vi "Configure CW Generation.vi"(0 "session in":T1[](array[typedef]) {"rx baseband session"."3630 session"."Address Space" items=["VXI/VME A16"=1, "VXI/VME A24"=2, "VXI/VME A32"=3, "VXI/VME A64"=4, "PXI Memory Allocations"=9, "PXI Configuration"=10, "PXI BAR0"=11, "PXI BAR1"=12, "PXI BAR2"=13, "PXI BAR3"=14, "PXI BAR4"=15, "PXI BAR5"=16]; "tx baseband session"."3610 session"."Address Space" items=["VXI/VME A16"=1, "VXI/VME A24"=2, "VXI/VME A32"=3, "VXI/VME A64"=4, "PXI Memory Allocations"=9, "PXI Configuration"=10, "PXI BAR0"=11, "PXI BAR1"=12, "PXI BAR2"=13, "PXI BAR3"=14, "PXI BAR4"=15, "PXI BAR5"=16]}, 5 "tone 1":cluster{"frequency (Hz)":dbl, "gain (dBFS)":dbl}={"frequency (Hz)"=0.0, "gain (dBFS)"=-inf} {"gain (dBFS)" format="%#_13g"; "frequency (Hz)" format="%#_13p"}, 7 "tone 2":cluster{"frequency (Hz)":dbl, "gain (dBFS)":dbl}={"frequency (Hz)"=0.0, "gain (dBFS)"=-inf} {"gain (dBFS)" format="%#_13g"; "frequency (Hz)" format="%#_13p"}, 9 "sample rate":dbl=3072000000.0 format="%#_13p", 11 "error in":errorcluster) -> (4 "session out":T1[](array[typedef]) {"rx baseband session"."3630 session"."Address Space" items=["VXI/VME A16"=1, "VXI/VME A24"=2, "VXI/VME A32"=3, "VXI/VME A64"=4, "PXI Memory Allocations"=9, "PXI Configuration"=10, "PXI BAR0"=11, "PXI BAR1"=12, "PXI BAR2"=13, "PXI BAR3"=14, "PXI BAR4"=15, "PXI BAR5"=16]; "tx baseband session"."3610 session"."Address Space" items=["VXI/VME A16"=1, "VXI/VME A24"=2, "VXI/VME A32"=3, "VXI/VME A64"=4, "PXI Memory Allocations"=9, "PXI Configuration"=10, "PXI BAR0"=11, "PXI BAR1"=12, "PXI BAR2"=13, "PXI BAR3"=14, "PXI BAR4"=15, "PXI BAR5"=16]}, 15 "error out":errorcluster)   [LabVIEW 2019]
uses:
  TypeDefs/Session.ctl
  <instrlib>/niMmWave/ni3620/Config/v1/Host/Public/High-Level/niMmWave Session.ctl
  <instrlib>/_niInstr/Register Bus/v0/Host/Public/Register Bus Session.ctl
  <instrlib>/_niInstr/Register Bus/v0/Host/Private/Session Data.ctl
  <instrlib>/niMmWave/ni3620/Config/v1/Host/Public/Typedefs/Board Information.ctl
  <instrlib>/niMmWave/ni3620/Config/v1/Host/Public/Typedefs/Hardware Revision.ctl
  <instrlib>/niMmWave/ni3620/Config/v1/Host/Public/Typedefs/Gain Mapping.ctl
  <instrlib>/niMmWave/ni3620/Config/v1/Host/Public/Typedefs/Correction Data.ctl
  <instrlib>/niMmWave/ni3620/Config/v1/Host/Public/Typedefs/Opera Characterization.ctl
  <instrlib>/niMmWave/ni3620/Config/v1/Host/Public/Corrections/Typedefs/Opera Characterization Main Header.ctl
  <instrlib>/niMmWave/ni3620/Config/v1/Host/Public/Corrections/Typedefs/Opera IF Board Information.ctl
  <instrlib>/niMmWave/ni3620/Config/v1/Host/Public/Corrections/Typedefs/Opera Characterization Instance Header.ctl
  <instrlib>/niMmWave/ni3620/Config/v1/Host/Public/Corrections/Typedefs/Opera Characterization Device Data Header.ctl
  <instrlib>/niMmWave/ni3620/Config/v1/Host/Public/Corrections/Typedefs/Opera LO Characterization Data Header.ctl
  <instrlib>/niMmWave/ni3620/Config/v1/Host/Public/Corrections/Typedefs/Opera IF Board Characterization Data Header.ctl
  <instrlib>/niMmWave/ni3620/Config/v1/Host/Public/Corrections/Typedefs/Opera Characterization Device Data.ctl
  <instrlib>/niMmWave/ni3620/Config/v1/Host/Public/Corrections/Typedefs/Opera LO2 Board Characterization Data.ctl
  <instrlib>/niMmWave/ni3620/Config/v1/Host/Public/Corrections/Typedefs/Opera LO Characterization Data.ctl
  <instrlib>/niMmWave/ni3620/Config/v1/Host/Public/Corrections/Typedefs/Opera IF Board Characterization Data.ctl
  <instrlib>/niMmWave/ni3620/Config/v1/Host/Public/Corrections/Typedefs/Opera IQ Impairment Data.ctl
  <instrlib>/niMmWave/ni3620/Config/v1/Host/Public/Typedefs/mmWave Adapter Session Data.ctl
  <instrlib>/niMmWave/ni3620/Config/v1/Host/Public/Typedefs/mmWave Adapter Data.ctl
  <instrlib>/niMmWave/ni3620/Config/v1/Host/Public/Typedefs/mmWave Adapter 2.ctl
  <instrlib>/niMmWave/ni3620/Config/v1/Shared/Typedefs/Subsystem ID.ctl
  <instrlib>/niMmWave/ni3620/Config/v1/Host/Public/Typedefs/mmWave Adapter Channel Information.ctl
  <instrlib>/niMmWave/ni3620/Config/v1/Host/Public/Typedefs/Temperature Coefficients.ctl
  <instrlib>/niMmWave/ni3620/Config/v1/Host/Public/Typedefs/mmWave Characterization.ctl
  <instrlib>/niMmWave/ni3620/Config/v1/Host/Public/Corrections/Typedefs/mmWave Characterization Main Header.ctl
  <instrlib>/niMmWave/ni3620/Config/v1/Host/Public/Corrections/Typedefs/mmWave Characterization Instance Header.ctl
  <instrlib>/niMmWave/ni3620/Config/v1/Host/Public/Typedefs/Session Cache.ctl
  <instrlib>/niMmWave/ni3620/Config/v1/Host/Public/Typedefs/LO2 settings cache.ctl
  <instrlib>/niMmWave/ni3620/Config/v1/Host/Public/Typedefs/LO2 source.ctl
  <instrlib>/niMmWave/ni3620/Config/v1/Host/Public/Typedefs/Desired and Coerced.ctl
  <instrlib>/niMmWave/ni3620/Config/v1/Host/Public/Typedefs/Export cache.ctl
  <instrlib>/niMmWave/ni3620/Config/v1/Host/Public/Typedefs/Path cache.ctl
  <instrlib>/niMmWave/ni3620/Config/v1/Host/Public/Typedefs/Daughterboard Type.ctl
  <instrlib>/niMmWave/ni3620/Config/v1/Host/Public/Typedefs/LO1 settings cache.ctl
  <instrlib>/niMmWave/ni3620/Config/v1/Host/Public/Typedefs/LO1 Source.ctl
  <instrlib>/niMmWave/ni3620/Config/v1/Host/Public/Typedefs/mmWave export cache.ctl
  <instrlib>/niMmWave/ni3620/Config/v1/Host/Private/Board/LO2/LO2 Board Configuration Cache.ctl
  <instrlib>/niMmWave/ni3620/Config/v1/Host/Public/Typedefs/reference clock routing settings.ctl
  <instrlib>/niMmWave/ni3620/Config/v1/Host/Public/Typedefs/LO2 routing settings.ctl
  <instrlib>/niMmWave/ni3620/Config/v1/Host/Private/Board/LO1/LO1 Board Configuration Cache.ctl
  <instrlib>/niMmWave/ni3620/Config/v1/Host/Public/Typedefs/LO1 source settings.ctl
  <instrlib>/niMmWave/ni3620/Config/v1/Host/Public/Typedefs/LO1 export settings.ctl
  <instrlib>/niMmWave/ni3620/Config/v1/Host/Public/Typedefs/LO1 mmWave settings.ctl
  TypeDefs/Tx Baseband Session.ctl
  <instrlib>/niMmWave/ni3610 and ni3630/controls/public/Main Settings.ctl
  <vilib>/Instr/_visa.llb/VISA Register Access Address Space.ctl
  <instrlib>/niMmWave/ni3610 and ni3630/controls/public/Register Adresses.ctl
  <instrlib>/niMmWave/ni3610 and ni3630/controls/public/Base Card Type.ctl
  <instrlib>/niMmWave/ni3610 and ni3630/controls/private/IQ Card Revision.ctl
  <instrlib>/niMmWave/ni3610 and ni3630/controls/public/Board Capability.ctl
  TypeDefs/Blank FPGA Reference.ctl
  TypeDefs/Rx Baseband Session.ctl
  TypeDefs/Hardware Configuration.ctl
  TypeDefs/Direction.ctl
  TypeDefs/Gain Ranging.ctl
  TypeDefs/PXI Trigger Bus Info.ctl
  TypeDefs/TX FPGA Reference.ctl
  <vilib>/Utility/error.llb/Error Cluster From Error Code.vi
  <vilib>/rvi/errors/niLvFpgaAdjustHostInterfaceError.vi
  <vilib>/rvi/interface/nirviReadWriteControl/nirviReadWriteControl.xnode
  mmWave HW Control/mmWave HW Control.lvlib
  NiFpgaLv.dll
  <vilib>/rvi/interface/Simulation/niFpgaSimulationCallBeginRW.vi
  <instrlib>/niMmWave/ni3620/Config/v1/Host/niMmWave Config v1 Host.lvlib
  <instrlib>/niMmWave/ni3620/Config/v1/Shared/niMmWave Config v1 Shared.lvlib
  <instrlib>/_niInstr/Register Bus/v0/Host/niInstr Register Bus v0 Host.lvlib
  <instrlib>/niMmWave/ni3610 and ni3630/ni3610_and_ni3630_Driver_Lib.lvlib
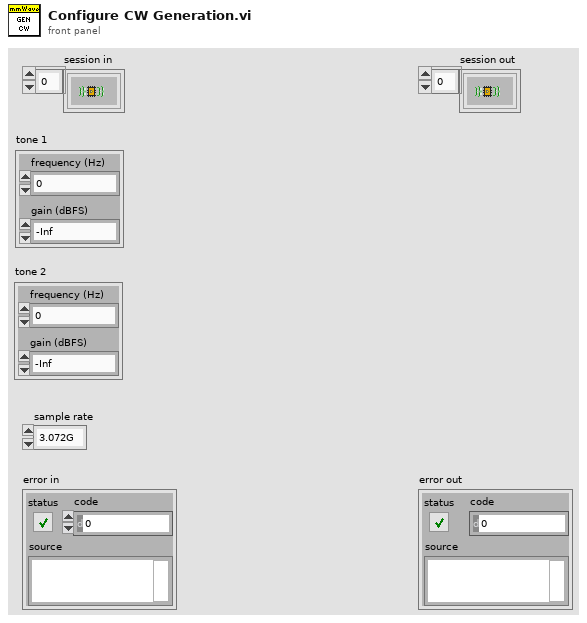
[diagram p1: front panel]
types:
  T1 = typedef "Session.ctl" = cluster{"3620 session":refnum<queue>, "tx baseband session":T2, "rx baseband session":T10, "tx gain (dB)":dbl, "rx gain (dB)":dbl, "hardware configuration":T11, "gain ranging":T13[], "pxi trigger bus information":T14}
  T2 = typedef "Tx Baseband Session.ctl" = cluster{"3610 session":T3, "7902 reference":T9}
  T3 = typedef "ni3610_and_ni3630_Driver_Lib.lvlib/Main Settings.ctl" = cluster{"VISA resource name":refnum<visa-resource-name>, "Address Space":T4, "window_offset":u32, "register_addresses":T5, "required_MM_fpga_version":cluster{"signature":u32, "hardware":u32, "current revision":u32, "oldest revision":u32}, "CPLD Oldest Compat Version ":cluster{"hardware":u32, "CPLD firmware":u32}, "MM_FPGA_image_location":string, "is_init":bool, "card_type":T6, "DacLmkConfigFileName":string, "AdcLmkConfigFileName":string, "AdcConfigFileName":string, "DacConfigFileName_RevA":string, "DacConfigFileName_RevB":string, "Mulde hardware revision":u8, "bypass DAC PLL\n":bool, "IQ Card Revision":T7, "board capability":T8}
  T4 = typedef "VISA Register Access Address Space.ctl" = u16
  T5 = typedef "ni3610_and_ni3630_Driver_Lib.lvlib/Register Adresses.ctl" = cluster{"MM based Registers":cluster{"Revision":u32, "OldestCompatRev":u32, "signature":u32, "scratch":u32, "LedControl":u32, "BoardHwRev":u32, "BoardControl":u32, "ThermalStatus":u32, "BasebandStatus":u32, "BasebandControl":u32, "BasebandAuxSetup":u32, "BasebandAuxStatus":u32, "LmkSyncOutSetup":u32, " AdcSyncOutSetup":u32, " InjSyncOutSetup":u32, " PxiTrig0OutSetup":u32, " PxiTrig1OutSetup":u32, " PxiTrig2OutSetup":u32, " PxiTrig3OutSetup":u32, " PxiTrig4OutSetup":u32, " PxiTrig5OutSetup":u32, " PxiTrig6OutSetup":u32, " PxiTrig7OutSetup":u32}, "CPLD based Registers":cluster{"SlaveSignature":u32, "SlaveRevision":u32, "SlaveOldestCompatRev":u32, "SlaveScratch":u32, "SlaveSetup":u32, "SlaveStatus":u32, "IDacReg_offset":u32, "LMKRegGrp0_offset":u32, "QDacReg_offset":u32, "BrdTempSensorVal":u32, "TempSensorPowerDown":u32, "GPIOReg_offset":u32, "IAdcReg_offset":u32, "QAdcReg_offset":u32, "LMKRegGrp1_offset":u32, "QadcTempSensorVal":u32, "IadcTempSensorVal":u32, "RevisionReg":u32, "VcxoReg":u32, "CpldStatusReg":u32, "PowerReg":u32, "VBiasEnReg":u32, "ExtRefOeReg":u32, "QdacCtrlReg":u32, "QdacStatusReg":u32, "IdacCtrlReg":u32, "IdacStatusReg":u32, "QdacJtagIn":u32, "QdacJtagOut":u32, "IdacJtagIn":u32, "IdacJtagOut":u32, "IqDcSetupReg":u32, "QadcStatusReg":u32, "IadcStatusReg":u32, "BrdSetupReg":u32, "IqDcRevisionReg":u32, "PllStatusReg":u32, "EndpointScratchReg":u32, "AdcSyncCfgReg":u32, "IqCardOpampReg":u32}, "CPLD Register Offset":u32, "MM  Register Offset":u32, " PxiTrig0OutSetup":u32}
  T6 = typedef "ni3610_and_ni3630_Driver_Lib.lvlib/Base Card Type.ctl" = enum16{"unspecified", "ADC", "DAC"}
  T7 = typedef "ni3610_and_ni3630_Driver_Lib.lvlib/IQ Card Revision.ctl" = enum16{"RevA", "RevB", "RevC", "RevD"}
  T8 = typedef "ni3610_and_ni3630_Driver_Lib.lvlib/Board Capability.ctl" = cluster{"baseband sync":enum16{"no baseband sync", "baseband sync"}}
  T9 = typedef "Blank FPGA Reference.ctl" = refnum<k20>
  T10 = typedef "Rx Baseband Session.ctl" = cluster{"3630 session":T3, "7902 reference":T9}
  T11 = typedef "Hardware Configuration.ctl" = cluster{"direction":T12, "baseband only":bool}
  T12 = typedef "Direction.ctl" = enum16{"Transceiver", "Receiver", "Transmitter"}
  T13 = typedef "Gain Ranging.ctl" = cluster{"gain ranging active scope":string, "gain ranging stream session":refnum<k20>}
  T14 = typedef "PXI Trigger Bus Info.ctl" = cluster{"chassis resource name":refnum<visa-resource-name>, "7902R (TX)":i16, "3610 (TX)":i16, "3620 (IF)":i16, "3630 (RX)":i16, "7902R (RX)":i16}
  T15 = cluster{"frequency (Hz)":dbl, "gain (dBFS)":dbl}[]
  T16 = cluster{"I":cluster{"tone 1":bool, "tone 2":bool}, "Q":cluster{"tone 1":bool, "tone 2":bool}}
  T17 = typedef "TX FPGA Reference.ctl" = refnum<k20>
  T18 = cluster{"frequency":fxp<+/-,48,0>, "gain":fxp<+/-,18,1>, "phase":fxp<+/-,21,0>, "offset":cluster{"offset I":fxp<+/-,18,1>, "offset Q":fxp<+/-,18,1>}}
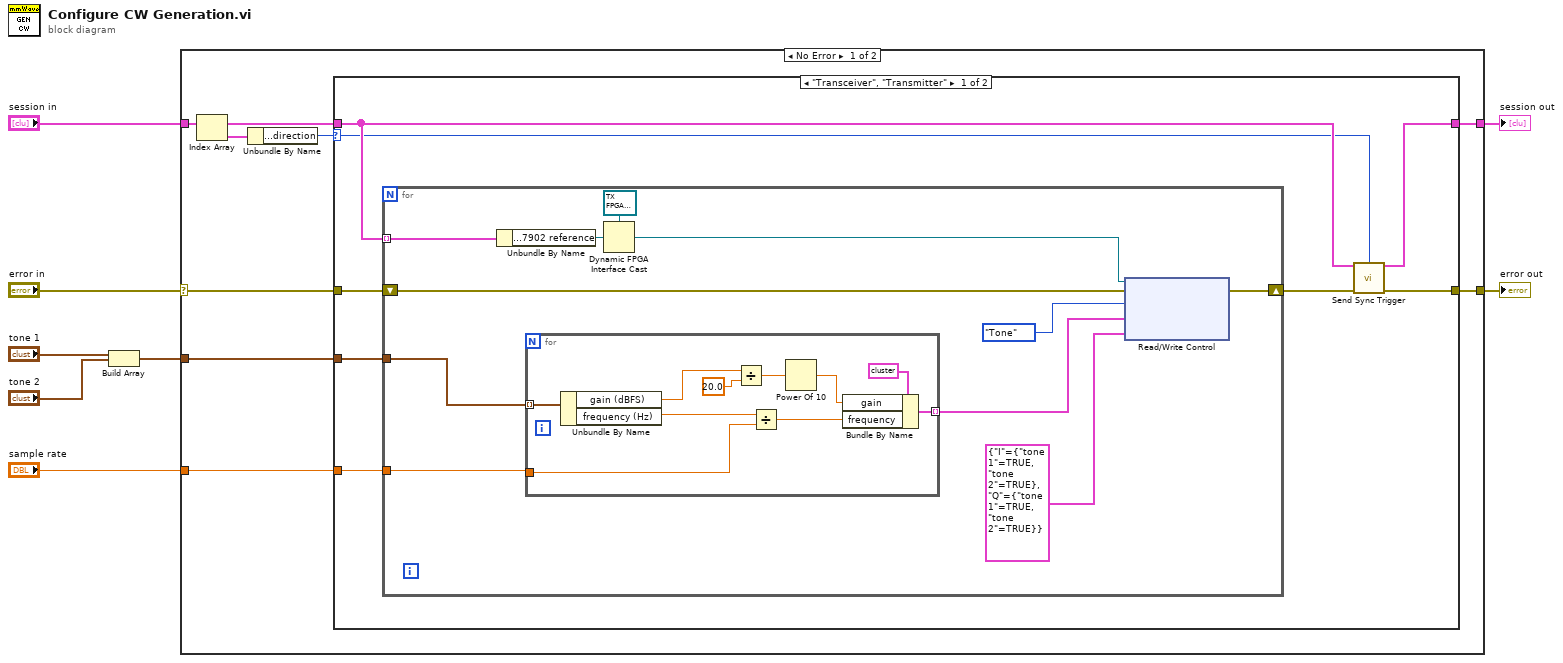
[diagram p0: block diagram]
diagram:
  n1 = Build Array("tone 1", "tone 2") -> (w1:T15)
  n2 = case shown="No Error" "error in" {
    selector: "error in" -> [w16 w49]
    tunnel: "session in" -> [w14 w48]
    tunnel: [w15 w49] -> w7
    tunnel: [w11 w48] -> w5
    tunnel: "sample rate" -> [w10 _]
    tunnel: w1 -> [w9 _]
    frame No Error {
      n3 = Index Array(array=w14) -> (element=w13:T1)  [unwired: 1 in]
      n4 = Unbundle By Name(w13) -> ("hardware configuration.direction"=w12:T12)
      n5 = case shown="\"Transceiver\", \"Transmitter\"" w12 {
        selector: w12 -> [w17 _]
        tunnel: w16 -> [w24 w47]
        tunnel: [w22 w47] -> w15
        tunnel: w14 -> [w21 w46]
        tunnel: [w20 w46] -> w11
        tunnel: w10 -> [w19 _]
        tunnel: w9 -> [w18 _]
        frame "Transceiver", "Transmitter" {
          n6 = for {
            shift-right: [w33] -> w23
            shift-left: w24 -> [w32]
            tunnel: w21 -> [w31] mode=indexing
            tunnel: w19 -> [w27]
            tunnel: w18 -> [w28]
            n7 = Unbundle By Name(w31) -> ("tx baseband session.7902 reference"=w30:T9)
            n8 = for {
              tunnel: w28 -> [w45] mode=indexing
              tunnel: w27 -> [w44]
              tunnel: [w40] -> w26 mode=indexing
              n9 = Unbundle By Name(w45) -> ("gain (dBFS)"=w37:dbl, "frequency (Hz)"=w43:dbl)
              n10 = Divide(x=w37, y=20.0) -> (x/y=w38:dbl)
              n11 = Divide(x=w43, y=w44) -> (x/y=w41:dbl)
              n12 = Power Of 10(x=w38) -> (10^x=w36:dbl)
              n13 = Bundle By Name(cluster=T18 {"frequency"=0.0, "gain"=0.9999923706054688, "phase"=0.0, "offset"={"offset I"=0.0, "offset Q"=0.0}} ("element"), "gain"=w36, "frequency"=w41) -> (w40:T18)
            }
            n14 = Dynamic FPGA Interface Cast(Session In=T17 refnum ("Refnum in"), Type=w30) -> (Session Out=w34:T17)
            n15 = xnode "Read/Write Control"("FPGA VI Reference In"=w34, "error in"=w32, "waveform type"=enum16{"Tone", "Waveform Generation", "Pulse"}."Tone", "tone.parameters"=w26, "tone.routing"=T16 {"I"={"tone 1"=TRUE, "tone 2"=TRUE}, "Q"={"tone 1"=TRUE, "tone 2"=TRUE}}) -> ("error out"=w33:errorcluster)  [unwired: 1 out]
          }
          n16 = call "Send Sync Trigger.vi"("session in"=w21, "sync select"=w17, "error in"=w23) -> ("session out"=w20:T1[], "error out"=w22:errorcluster)  [unwired: 11 in]
        }
        frame "Receiver" {
        }
      }
    }
    frame Error {
    }
  }
  "session out" <- w5
  "error out" <- w7
